vi "9229_UI.vi"(8 "error in (no error)":errorcluster, 11 "Node Ptr":T2 format="%.0x") -> (0 "error out":errorcluster)   [LabVIEW 2011, in "Modules.lvlib" / "9229.lvclass"]
uses:
  9229.lvclass
  <vilib>/NI Veristand/Custom Device API/Custom Device Item Ref.ctl
  RSI Module/SubPanel Command.ctl
  Data rate.ctl
  9229.lvclass/9229.ctl
  RSI Module/RSI Module.lvclass
  <vilib>/NI Veristand/Custom Device API/Custom Device API.lvlib
panel:
  in  "ADC sampling rate":T1 items=["50.000 kS/s", "25.000 kS/s", "16.667 kS/s", "12.500 kS/s", "10.000 kS/s", "8.333 kS/s", "7.143 kS/s", "6.250 kS/s", "5.556 kS/s", "5.000 kS/s", "4.545 kS/s", "4.167 kS/s", "3.846 kS/s", "3.571 kS/s", "3.333 kS/s", "3.125 kS/s", "2.941 kS/s", "2.778 kS/s", "2.632 kS/s", "2.500 kS/s", "2.381 kS/s", "2.273 kS/s", "2.174 kS/s", "2.083 kS/s", "2.000 kS/s", "1.923 kS/s", "1.852 kS/s", "1.786 kS/s", "1.724 kS/s", "1.667 kS/s", "1.613 kS/s"]
  in  "SubPanel Event":refnum<user-event>
  in  "Header":cluster{"Section Name":string}={"Section Name"="NI 9205 Settings"}
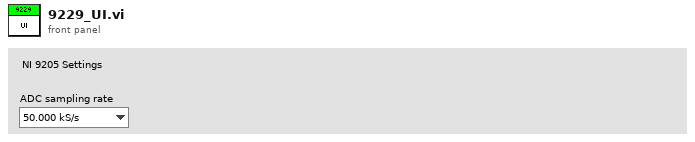
[diagram p1: front panel]
types:
  T1 = typedef "Modules.lvlib/9229.lvclass/Data rate.ctl" = u32
  T2 = typedef "Custom Device API.lvlib/Custom Device Item Ref.ctl" = u64
  T3 = typedef "Modules.lvlib/RSI Module.lvclass/Module Models.ctl" = enum16{"Empty", "NI 9201", "NI 9203", "NI 9205", "NI 9206", "NI 9207", "NI 9208", "NI 9211", "NI 9213", "NI 9214", "NI 9215", "NI 9217", "NI 9219", "NI 9221", "NI 9225", "NI 9227", "NI 9229", "NI 9233", "NI 9234", "NI 9235", "NI 9236", "NI 9237", "NI 9239", "NI 9263", "NI 9264", "NI 9265", "NI 9269", "NI 9375", "NI 9401", "NI 9402", "NI 9403", "NI 9411", "NI 9421", "NI 9422", "NI 9423", "NI 9425", "NI 9426", "NI 9435", "NI 9472", "NI 9474", "NI 9475", "NI 9476", "NI 9477", "NI 9478", "NI 9481", "NI 9482", "NI 9485"}
  T4 = typedef "Modules.lvlib/RSI Module.lvclass/SubPanel Command.ctl" = enum16{"Stop"}
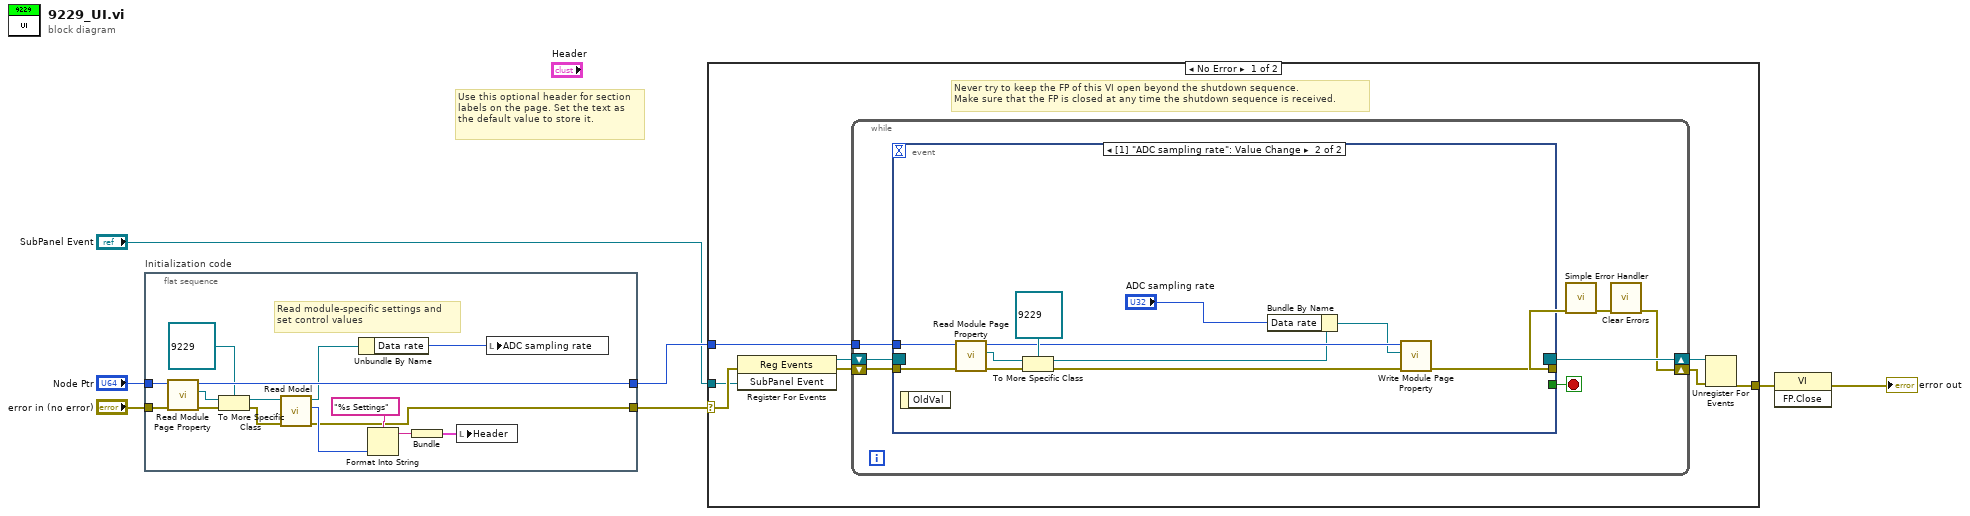
[diagram p0: block diagram]
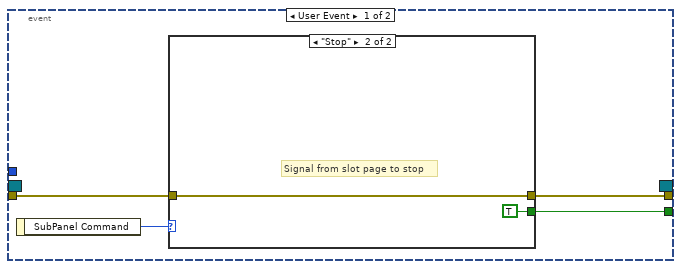
[diagram p2: hidden frame]
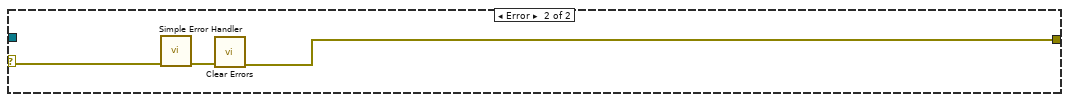
[diagram p4: hidden frame]
diagram:
  # "Use this optional header for section labels on the page. Set the text as the default value to store it."
  n1 = flat-sequence "Initialization code" {
    tunnel: "error in (no error)" -> [w21]
    tunnel: "Node Ptr" -> [w22]
    tunnel: [w9] -> w1
    tunnel: [w20] -> w4
    frame #0 {
      # "Read module-specific settings and\nset control values"
      n2 = call "Read Module Page Property.vi"("error in (no error)"=w21, "Node Ptr In"=w22) -> ("error out"=w19:errorcluster, "RSI Module"=w17:refnum<class "RSI Module.lvclass">, "Node Ptr Out"=w20:T2)  [unwired: 7 in]
      n3 = To More Specific Class(target class=refnum<class "9229.lvclass"> refnum ("9205 in"), reference=w17, error in=w19) -> (specific class reference=w16:refnum<class "9229.lvclass">, error out=w15:errorcluster)
      n4 = call "Read Model.vi"("error in (no error)"=w15, "RSI Module in"=w16) -> ("error out"=w9:errorcluster, "Model"=w13:T3, "RSI Module out"=w10:refnum<class "9229.lvclass">)  [unwired: 7 in]
      n5 = Unbundle By Name(w10) -> ("Data rate"=w8:T1)
      n6 = Format Into String(format string="%s Settings", w13) -> (resulting string=w11:string)  [unwired: 2 in, 1 out]
      n7 = Bundle(w11) -> (w14:cluster{string})  [unwired: 1 in]
      n8 = local write "Header"(w14) -> ()
      n9 = local write "ADC sampling rate"(w8) -> ()
    }
  }
  n10 = case shown="No Error" w1 {
    selector: w1 -> [w24 w59]
    tunnel: [w28 w57] -> w7
    tunnel: w4 -> [w25 _]
    tunnel: "SubPanel Event" -> [w23 _]
    frame No Error {
      # "Never try to keep the FP of this VI open beyond the shutdown sequence.\nMake sure that the FP is closed at any time the shutdown sequence is received."
      n11 = register-events(error in=w24, w23) -> (reference out=w26:refnum<event-registration>, error out=w27:errorcluster)  [unwired: 1 in]
      n12 = while {
        tunnel: w25 -> [w34]
        shift-right: [w31] -> w29
        shift-left: w27 -> [w37]
        shift-right: [w38] -> w30
        shift-left: w26 -> [w36]
        stop <- w35 stop-if-true
        n13 = event shown="[1] \"ADC sampling rate\": Value Change" {
          selector: w36 -> [_ _]
          dyn-events: [_ _] -> w38
          timeout: _ -> [_ _]
          tunnel: w37 -> [w41 w50]
          tunnel: [w40 _] -> w35
          tunnel: [w39 w49] -> w33
          tunnel: w34 -> [_ w51]
          event User Event {
            n14 = event-data() -> ("SubPanel Command"=w42:T4)  [unwired: 1 out]
            n15 = case shown="\"Stop\"" w42 {
              tunnel: w41 -> [w43 w44]
              tunnel: [w43 w44] -> w39
              tunnel: [_ TRUE] -> w40
              frame Default {
              }
              frame "Stop" {
                # "Signal from slot page to stop"
              }
            }
          }
          event Value Change {
            n16 = event-data() -> ()  [unwired: 2 out]
            n17 = call "Read Module Page Property.vi"("error in (no error)"=w50, "Node Ptr In"=w51) -> ("error out"=w54:errorcluster, "RSI Module"=w55:refnum<class "RSI Module.lvclass">, "Node Ptr Out"=w52:T2)  [unwired: 7 in]
            n18 = To More Specific Class(target class=refnum<class "9229.lvclass"> refnum ("9205 in"), reference=w55, error in=w54) -> (specific class reference=w48:refnum<class "9229.lvclass">, error out=w53:errorcluster)
            n19 = Bundle By Name(cluster=w48, "Data rate"="ADC sampling rate") -> (w47:refnum<class "9229.lvclass">)
            n20 = call "Write Module Page Property.vi"("error in (no error)"=w53, "RSI Module"=w47, "Node Ptr In"=w52) -> ("error out"=w49:errorcluster)  [unwired: 6 in, 2 out]
          }
        }
        n21 = call <vilib>:"Simple Error Handler.vi"("error in (no error)"=w33) -> ("error out"=w32:errorcluster)  [unwired: 1 in, 7 out]
        n22 = call <vilib>:"Clear Errors.vi"("error in (no error)"=w32) -> ("error out"=w31:errorcluster)  [unwired: 6 out]
      }
      n23 = Unregister For Events(event registration refnum=w30, error in=w29) -> (error out=w28:errorcluster)
    }
    frame Error {
      n24 = call <vilib>:"Simple Error Handler.vi"("error in (no error)"=w59) -> ("error out"=w58:errorcluster)  [unwired: 1 in, 7 out]
      n25 = call <vilib>:"Clear Errors.vi"("error in (no error)"=w58) -> ("error out"=w57:errorcluster)  [unwired: 6 out]
    }
  }
  n26 = invoke class="VI" method="FP.Close"(error in=w7) -> (error out=→"error out":errorcluster)  [unwired: 2 in, 2 out]
